vi "算数平均滤波.vi"() -> ()   [LabVIEW 2018]
panel:
  in  "停止":bool
  out "数值":dbl
  in  "波形":dbl[](array[numeric])
  in  "采样数":dbl
  out "字符串":string="生成周期性随机噪声"
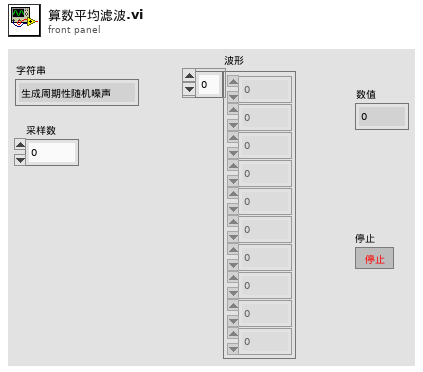
[diagram p1: front panel]
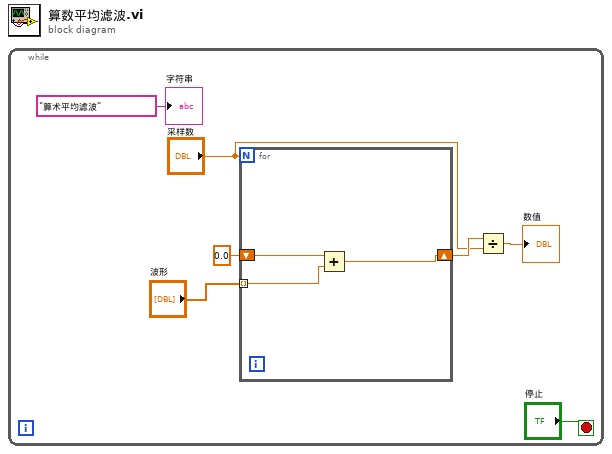
[diagram p0: block diagram]
diagram:
  n1 = while {
    stop <- "停止" stop-if-true
    n2 = for {
      N: "采样数" -> [_]
      shift-right: [w8] -> w4
      shift-left: 0.0 -> [w9]
      tunnel: "波形" -> [w10] mode=indexing
      n3 = Add(x=w9, y=w10) -> (x+y=w8:dbl)
    }
    n4 = Divide(x=w4, y="采样数") -> (x/y=→"数值":dbl)
    "字符串" <- "算术平均滤波"
  }
